vi "Read Config.vi"(10 "Config Path":path) -> (0 "Test Table":string[][](array[string]), 1 "C_Tol":dbl, 2 "P_Tol":dbl, 3 "PSID":dbl)   [LabVIEW 2018]
uses:
  <vilib>/Utility/config.llb/Read Key (Double).vi
  <vilib>/Utility/config.llb/Read Key (String).vi
  <vilib>/Utility/config.llb/NI_LVConfig.lvlib
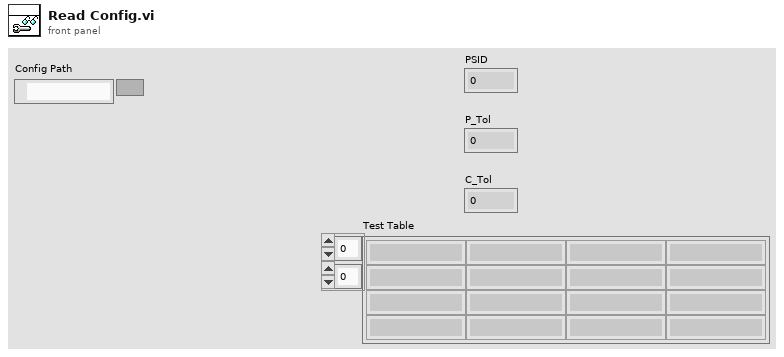
[diagram p1: front panel]
types:
  T1 = typedef "NI_LVConfig.lvlib/Config Data RefNum.ctl" = refnum<k1>
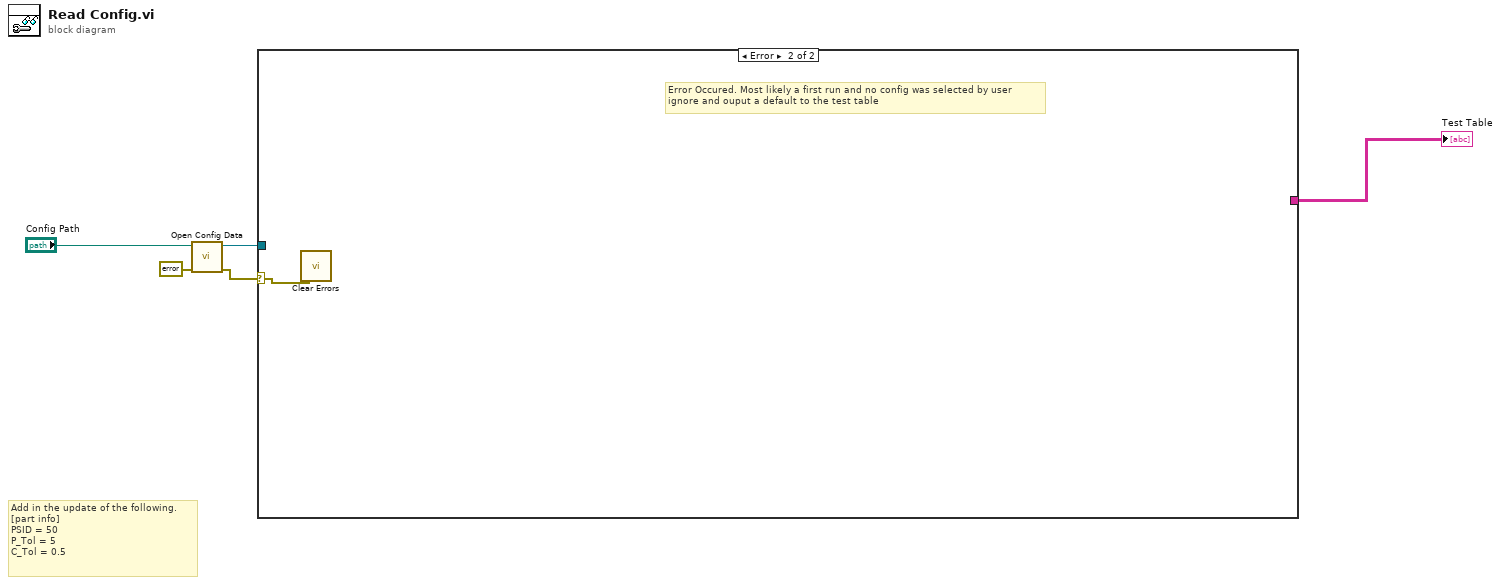
[diagram p0: block diagram]
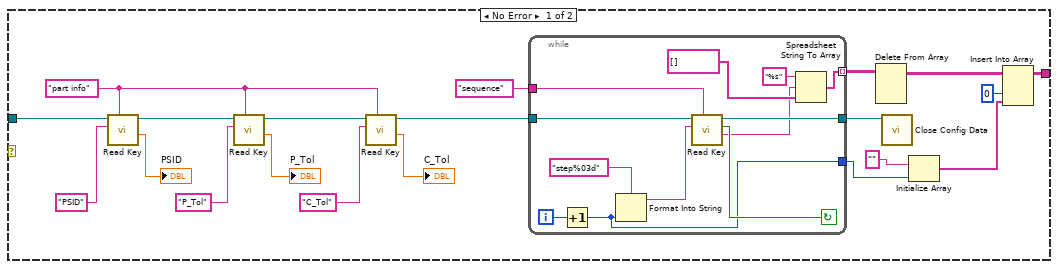
[diagram p2: hidden frame]
diagram:
  # "Add in the update of the following.\n[part info]\nPSID = 50\nP_Tol = 5\nC_Tol = 0.5"
  n1 = call <vilib>:"Open Config Data.vi"("error in (no error)"=errorcluster {"status"=FALSE, "code"=0, "source"=""}, "configuration file path"="Config Path") -> ("error out"=w2:errorcluster, "refnum"=w5:T1)  [unwired: 7 in, 1 out]
  n2 = case shown="Error" w2 {
    selector: w2 -> [_ w38]
    tunnel: w5 -> [w25 _]
    tunnel: [w10 _] -> w4
    frame No Error {
      w24 = "part info" ("section")
      n3 = call-poly <vilib>:"Read Key.vi"("section"=w24, "key"="PSID", "refnum"=w25) -> ("value"=→"PSID":dbl, "refnum out"=w17:T1)  [unwired: 5 in, 2 out]
      n4 = call-poly <vilib>:"Read Key.vi"("section"=w24, "key"="P_Tol", "refnum"=w17) -> ("value"=→"P_Tol":dbl, "refnum out"=w16:T1)  [unwired: 5 in, 2 out]
      n5 = call-poly <vilib>:"Read Key.vi"("section"=w24, "key"="C_Tol", "refnum"=w16) -> ("value"=→"C_Tol":dbl, "refnum out"=w15:T1)  [unwired: 5 in, 2 out]
      n6 = while {
        tunnel: w15 -> [w37]
        tunnel: "sequence" ("section") -> [w36]
        tunnel: [w31] -> w13
        tunnel: [w28] -> w12 mode=indexing
        tunnel: [w26] -> w9
        i -> [w35]
        stop <- w32 continue-if-true
        n7 = Increment(x=w35) -> (x+1=w26:i32)
        n8 = Format Into String(format string="step%03d", w26) -> (resulting string=w33:string)  [unwired: 2 in, 1 out]
        n9 = call-poly <vilib>:"Read Key.vi"("section"=w36, "key"=w33, "refnum"=w37) -> ("value"=w29:string, "found?"=w32:bool, "refnum out"=w31:T1)  [unwired: 5 in, 1 out]
        n10 = Spreadsheet String To Array(format string="%s", spreadsheet string=w29, array type (2D Dbl)=string[] []) -> (array=w28:string[])  [unwired: 1 in]
      }
      n11 = Delete From Array(array=w12) -> (array with subset deleted=w11:string[][])  [unwired: 3 in, 1 out]
      n12 = call <vilib>:"Close Config Data.vi"("refnum"=w13) -> ()  [unwired: 9 in, 2 out]
      n13 = Initialize Array("", w9) -> (w7:string[])
      n14 = Insert Into Array(array=w11, index (col)=0 ("disabled index (col)"), new element=w7) -> (w10:string[][])  [unwired: 1 in]
    }
    frame Error {
      # "Error Occured. Most likely a first run and no config was selected by user\nignore and ouput a default to the test table"
      n15 = call <vilib>:"Clear Errors.vi"("error in (no error)"=w38) -> ()  [unwired: 5 in, 2 out]
    }
  }
  "Test Table" <- w4
